vi "TagSetPixel.vi"(6 "Number of Bits":i32, 7 "Pixel Type Map":u8[][](array[numeric]), 8 "y":i32, 9 "x":i32, 10 "Code in":i64, 11 "Pixels in":T1[][](array[typedef])) -> (2 "Code out":i64, 3 "Pixels out":T1[][](array[typedef]))   [LabVIEW 2020, in "g_ar_toolkit.feature_detection.lvlib"]
uses:
  g_ar_toolkit.feature_detection.lvlib
  TagPixelType.ctl
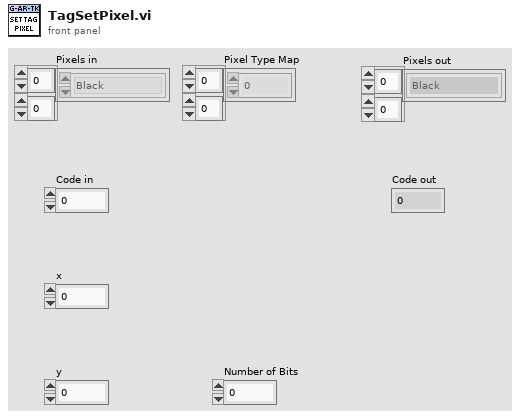
[diagram p1: front panel]
types:
  T1 = typedef "g_ar_toolkit.feature_detection.lvlib/TagPixelType.ctl" = enum8{"Black", "White", "Transparent"}
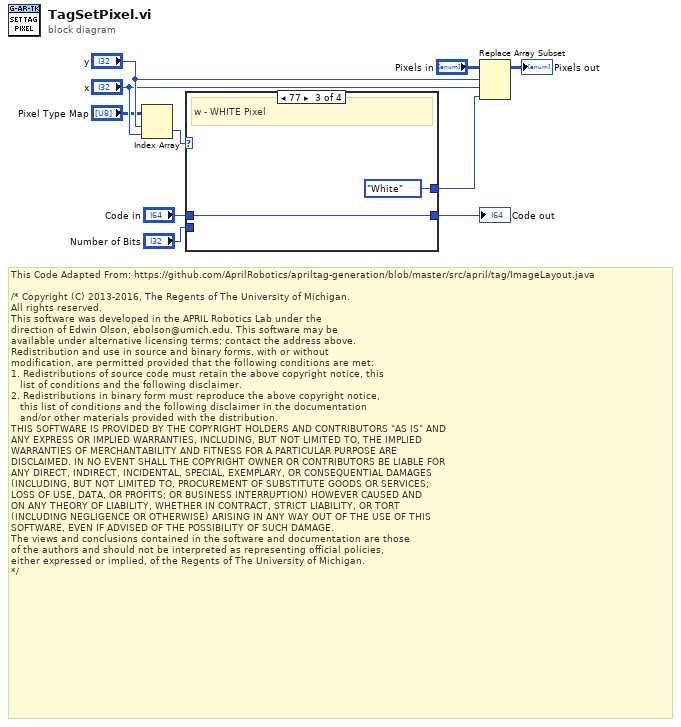
[diagram p0: block diagram]
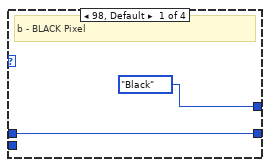
[diagram p2: hidden frame]
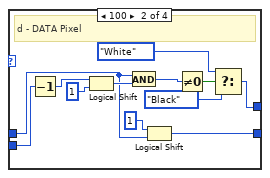
[diagram p3: hidden frame]
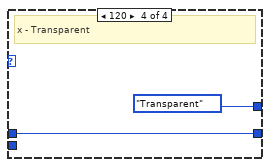
[diagram p4: hidden frame]
diagram:
  # "This Code Adapted From: https://github.com/AprilRobotics/apriltag-generation/blob/master/src/april/tag/ImageLayout.java\n\n/* Copyright (C) 2013-2016, The Regents of The University of Michigan.\nAll rights reserved.\nThis software was developed in the APRIL Robotics Lab under the\ndirection of Edwin Olson, ebolson@umich.edu. This software may be\navailable under alternative licensing terms; contact the address above.\nRedistribution and use in source and binary forms, with or without\nmodification, are permitted provided that the following conditions are met:\n1. Redistributions of source code must retain the above copyright notice, this\n   list of conditions and the following disclaimer.\n2. Redistributions in binary form must reproduce the above copyright notice,\n   this list of conditions and the following disclaimer in the documentation\n   and/or other materials provided with the distribution.\nTHIS SOFTWARE IS PROVIDED BY THE COPYRIGHT HOLDERS AND CONTRIBUTORS \"AS IS\" AND\nANY EXPRESS OR IMPLIED WARRANTIES, INCLUDING, BUT NOT LIMITED TO, THE IMPLIED\nWARRANTIES OF MERCHANTABILITY AND FITNESS FOR A PARTICULAR PURPOSE ARE\nDISCLAIMED. IN NO EVENT SHALL THE COPYRIGHT OWNER OR CONTRIBUTORS BE LIABLE FOR\nANY DIRECT, INDIRECT, INCIDENTAL, SPECIAL, EXEMPLARY, OR CONSEQUENTIAL DAMAGES\n(INCLUDING, BUT NOT LIMITED TO, PROCUREMENT OF SUBSTITUTE GOODS OR SERVICES;\nLOSS OF USE, DATA, OR PROFITS; OR BUSINESS INTERRUPTION) HOWEVER CAUSED AND\nON ANY THEORY OF LIABILITY, WHETHER IN CONTRACT, STRICT LIABILITY, OR TORT\n(INCLUDING NEGLIGENCE OR OTHERWISE) ARISING IN ANY WAY OUT OF THE USE OF THIS\nSOFTWARE, EVEN IF ADVISED OF THE POSSIBILITY OF SUCH DAMAGE.\nThe views and conclusions contained in the software and documentation are those\nof the authors and should not be interpreted as representing official policies,\neither expressed or implied, of the Regents of The University of Michigan.\n*/"
  n1 = Index Array(array="Pixel Type Map", index (row)="y", index (col)="x") -> (element=w2:u8)
  n2 = case shown="77" w2 {
    tunnel: [TagPixelType."Black" ("TagPixelType") w16 TagPixelType."White" ("TagPixelType") TagPixelType."Transparent" ("TagPixelType")] -> w8
    tunnel: "Number of Bits" -> [_ w21 _ _]
    tunnel: "Code in" -> [w12 w19 w26 w28]
    tunnel: [w12 w22 w26 w28] -> w6
    frame 98, Default {
      # "b - BLACK Pixel"
    }
    frame 100 {
      # "d - DATA Pixel"
      n3 = Decrement(x=w21) -> (x-1=w15:i32)
      n4 = Logical Shift(y=w15, x=i64 1) -> (x << y=w24:i64)
      n5 = And(x=w19, y=w24) -> (x .and. y?=w23:i64)
      n6 = Logical Shift(y=i16 1, x=w19) -> (x << y=w22:i64)
      n7 = Not Equal To 0?(x=w23) -> (x != 0?=w17:bool)
      n8 = Select(t=TagPixelType."White" ("TagPixelType"), s=w17, f=TagPixelType."Black") -> (s? t:f=w16:T1)
    }
    frame 119 {
      # "w - WHITE Pixel"
    }
    frame 120 {
      # "x - Transparent"
    }
  }
  "Code out" <- w6
  n9 = Replace Array Subset(array="Pixels in", new element=w8, index (row)="y", index (col)="x") -> (→"Pixels out":T1[][])
